vi "Combine Waveforms.vi"(10 "Matrix of Carriers":T1) -> (2 "Combined Output":cdb[](array[numeric]))   [LabVIEW 2018]
uses:
  <vilib>/silver_ctls/ArrayMatrixCluster/Complex Matrix NI_Silver.ctl
  <vilib>/Analysis/Matrix/Numeric/Conversions/Matrix To Array - CM.vi
  <vilib>/Analysis/Matrix/NI_Matrix.lvlib
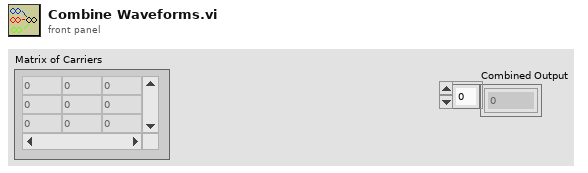
[diagram p1: front panel]
types:
  T1 = typedef "Complex Matrix NI_Silver.ctl" = cdb[][]
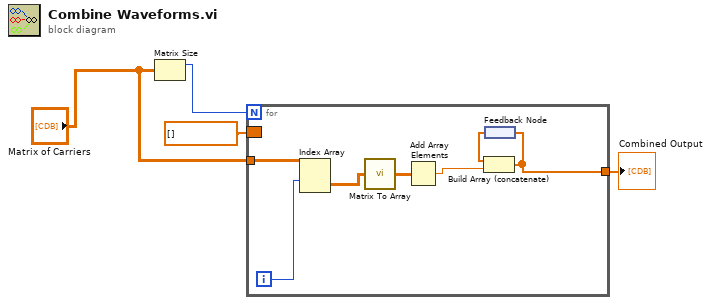
[diagram p0: block diagram]
diagram:
  n1 = Matrix Size(0:"Matrix of Carriers") -> (1:w4:i32)  [unwired: 1 out]
  n2 = for {
    N: w4 -> [_]
    tunnel: "Matrix of Carriers" -> [w11]
    border: cdb[] [] -> [_]
    tunnel: [w5] -> w1
    i -> [w10]
    n3 = Index Array(array=w11, index (row)=w10) -> (element=w9:T1)  [unwired: 1 in]
    n4 = call-poly <vilib>:"Matrix To Array.vi"("Complex Matrix"=w9) -> ("Complex 2D Array"=w8:cdb[][])
    n5 = Add Array Elements(numeric array=w8) -> (sum=w7:cdb)
    n6 = feedback #1() -> (w6:cdb[])
    n7 = Build Array (concatenate)(w6, w7) -> (w5:cdb[])
    n8 = feedback-in #1(w5) -> ()
  }
  "Combined Output" <- w1
